vi "RAW.vi"() -> ()   [LabVIEW 2017]
uses:
  <vilib>/registry/registry.llb/Registry RtKey.ctl
  <vilib>/registry/registry.llb/Write Registry Value Simple STR.vi
  <vilib>/registry/registry.llb/Read Registry Value Simple STR.vi
panel:
  out "error out":errorcluster
  in  "error in (no error)":errorcluster
  in  "stop":bool
  in  "TILL DATE":timestamp
  out "date/time string":string
  out "Sample Key Read?":bool
  out "Sample Key Written?":bool
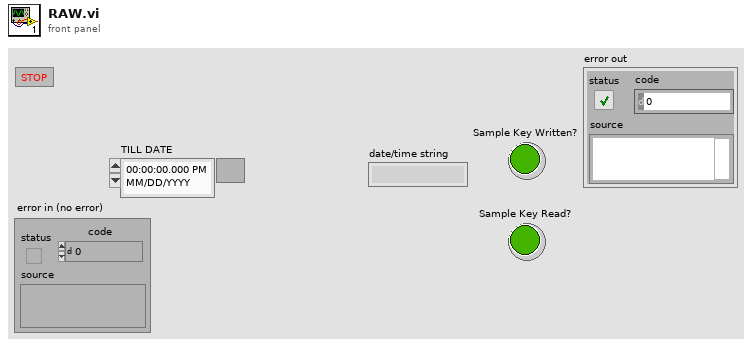
[diagram p1: front panel]
types:
  T1 = typedef "Registry RtKey.ctl" = enum32{"HKEY_CLASSES_ROOT", "HKEY_CURRENT_USER", "HKEY_LOCAL_MACHINE", "HKEY_USERS", "HKEY_PERFORMANCE_DATA", "HKEY_CURRENT_CONFIG", "HKEY_DYN_DATA"}
  T2 = typedef "Registry refnum.ctl" = refnum<k1>
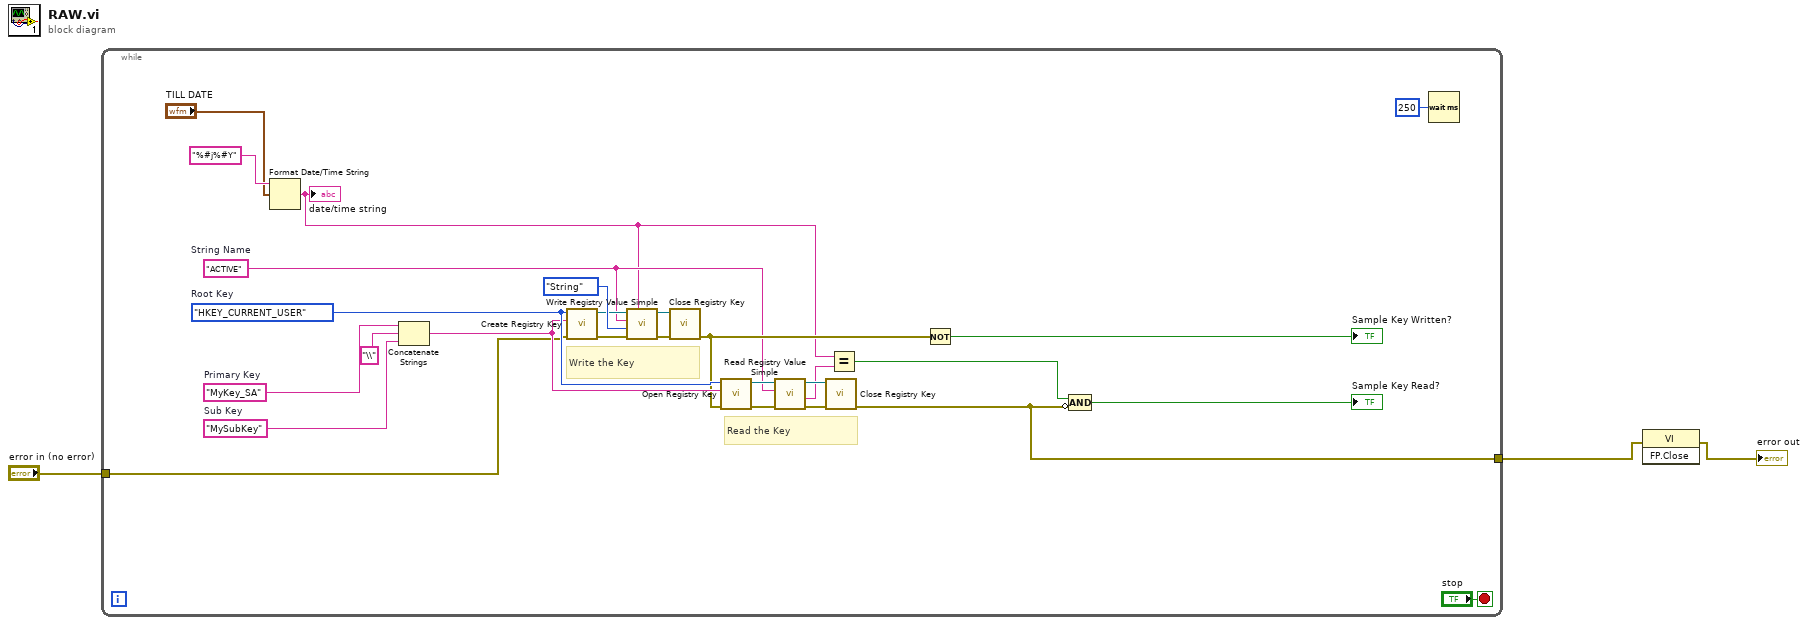
[diagram p0: block diagram]
diagram:
  n1 = while {
    tunnel: [w6] -> w2
    tunnel: "error in (no error)" -> [w5]
    stop <- "stop" stop-if-true
    w19 = "MySubKey"  # Sub Key
    w12 = "MyKey_SA"  # Primary Key
    w16 = "ACTIVE"  # String Name
    w21 = Registry_RtKey."HKEY_CURRENT_USER"  # Root Key
    # "Read the Key"
    # "Write the Key"
    n2 = Format Date/Time String(time format string (%c)="%#j%#Y", seconds (now)="TILL DATE") -> (date/time string=w9:string)  [unwired: 1 in]
    "date/time string" <- w9
    n3 = Concatenate Strings(w12, "\\", w19) -> (w20:string)
    n4 = call <vilib>:"Create Registry Key.vi"("error in (no error)"=w5, "subkey"=w20, "root key (HKEY_LOCAL_MACHINE)"=w21) -> ("error out"=w28:errorcluster, "refnum out"=w26:T2)  [unwired: 6 in, 1 out]
    n5 = call-poly <vilib>:"Write Registry Value Simple.vi"("String/Binary data"=w9, "error in (no error)"=w28, "simple data type"=enum16{"String", "Binary", "DWORD"}."String", "value"=w16, "refnum"=w26) -> ("error out"=w30:errorcluster, "refnum out"=w29:T2)  [unwired: 3 in]
    n6 = call <vilib>:"Close Registry Key.vi"("error in (no error)"=w30, "refnum"=w29) -> ("error out"=w18:errorcluster)  [unwired: 5 in]
    n7 = call <vilib>:"Open Registry Key.vi"("error in (no error)"=w18, "subkey"=w20, "root key (HKEY_LOCAL_MACHINE)"=w21) -> ("error out"=w22:errorcluster, "refnum out"=w23:T2)  [unwired: 7 in]
    n8 = call-poly <vilib>:"Read Registry Value Simple.vi"("error in (no error)"=w22, "value"=w16, "refnum"=w23) -> ("error out"=w25:errorcluster, "String/Binary data"=w15:string, "refnum out"=w24:T2)  [unwired: 3 in, 1 out]
    n9 = call <vilib>:"Close Registry Key.vi"("error in (no error)"=w25, "refnum"=w24) -> ("error out"=w6:errorcluster)  [unwired: 5 in]
    n10 = Equal?(x=w9, y=w15) -> (x = y?=w14:bool)
    n11 = Not(x=w18) -> (.not. x?=→"Sample Key Written?":bool)
    n12 = Compound Arithmetic op=AND(w14, invert w6) -> (→"Sample Key Read?":bool)
    n13 = Wait (ms)(milliseconds to wait=u32 250) -> ()  [unwired: 1 out]
  }
  n14 = invoke class="VI" method="FP.Close"(error in=w2) -> (error out=→"error out":errorcluster)  [unwired: 2 in, 2 out]
